vi "数据解码.vi"(11 "数组":u16[](array[numeric]) format="%04xH") -> (3 "读取值":T1 {"累积流量单位" items=["L", "M3", "T", "USG"]; "瞬时流量单位" items=["L/S", "L/M", "L/H", "M3/S", "M3/M", "M3/H", "T/S", "T/M", "T/H", "GPS", "GPM", "GPH"]})   [LabVIEW 2016, in "流量计集成.lvlib" / "MGG-KL-QC流量计.lvlib"]
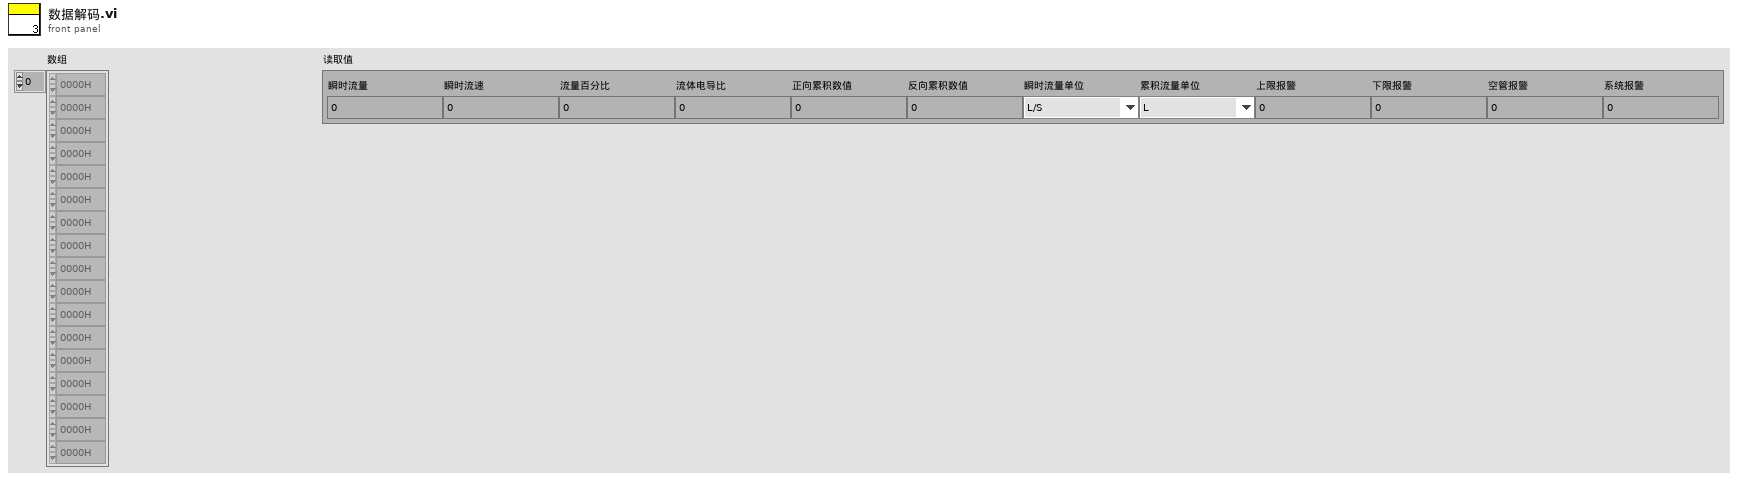
[diagram p1: front panel]
types:
  T1 = typedef "流量计集成.lvlib/MGG-KL-QC流量计.lvlib/读取值.ctl" = cluster{"瞬时流量":sgl, "瞬时流速":sgl, "流量百分比":sgl, "流体电导比":sgl, "正向累积数值":sgl, "反向累积数值":sgl, "瞬时流量单位":T2, "累积流量单位":T3, "上限报警":u16, "下限报警":u16, "空管报警":u16, "系统报警":u16}
  T2 = typedef "流量计集成.lvlib/MGG-KL-QC流量计.lvlib/瞬时流量单位.ctl" = u16
  T3 = typedef "流量计集成.lvlib/MGG-KL-QC流量计.lvlib/累积流量单位.ctl" = u16
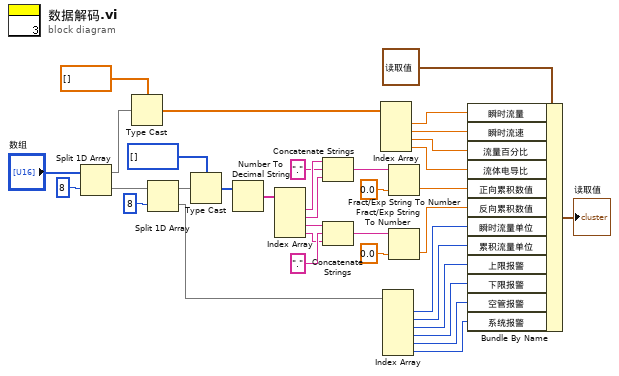
[diagram p0: block diagram]
diagram:
  n1 = Split 1D Array(array="数组", index=8 ("索引")) -> (first subarray=w1:u16[], second subarray=w34:u16[])
  n2 = Type Cast(type=sgl[] [], x=w1) -> (*(type *) &x=w15:sgl[])
  n3 = Split 1D Array(array=w34, index=8 ("索引")) -> (first subarray=w30:u16[], second subarray=w8:u16[])
  n4 = Type Cast(type=u32[] [], x=w30) -> (*(type *) &x=w29:u32[])
  n5 = Number To Decimal String(number=w29) -> (decimal integer string=w28:string[])  [unwired: 1 in]
  n6 = Index Array(array=w28) -> (element #1=w27:string, element #2=w26:string, element #3=w23:string, element #4=w22:string)  [unwired: 4 in]
  n7 = Concatenate Strings(w27, "." ("字符串"), w26) -> (w21:string)
  n8 = Concatenate Strings(w23, "." ("字符串"), w22) -> (w20:string)
  n9 = Index Array(array=w15) -> (element #1=w14:sgl, element #2=w13:sgl, element #3=w12:sgl, element #4=w11:sgl)  [unwired: 4 in]
  n10 = Index Array(array=w8) -> (element #1=w7:u16, element #2=w6:u16, element #3=w5:u16, element #4=w4:u16, element #5=w3:u16, element #6=w2:u16)  [unwired: 6 in]
  n11 = Fract/Exp String To Number(string=w21, default (0 dbl)=sgl 0.0 ("默认(0 DBL)")) -> (number=w10:sgl)  [unwired: 2 in, 1 out]
  n12 = Fract/Exp String To Number(string=w20, default (0 dbl)=sgl 0.0 ("默认(0 DBL)")) -> (number=w9:sgl)  [unwired: 2 in, 1 out]
  n13 = Bundle By Name(cluster=T1 {"瞬时流量"=0.0, "瞬时流速"=0.0, "流量百分比"=0.0, "流体电导比"=0.0, "正向累积数值"=0.0, "反向累积数值"=0.0, "瞬时流量单位"=0, "累积流量单位"=0, "上限报警"=0, "下限报警"=0, "空管报警"=0, "系统报警"=0} ("读取值"), "瞬时流量"=w14, "瞬时流速"=w13, "流量百分比"=w12, "流体电导比"=w11, "正向累积数值"=w10, "反向累积数值"=w9, "瞬时流量单位"=w7, "累积流量单位"=w6, "上限报警"=w5, "下限报警"=w4, "空管报警"=w3, "系统报警"=w2) -> (→"读取值":T1)
